vi "TL error.vi"(8 "error in (no error)":errorcluster, 11 "Return Code":i32) -> (0 "error out":errorcluster)   [LabVIEW 2014]
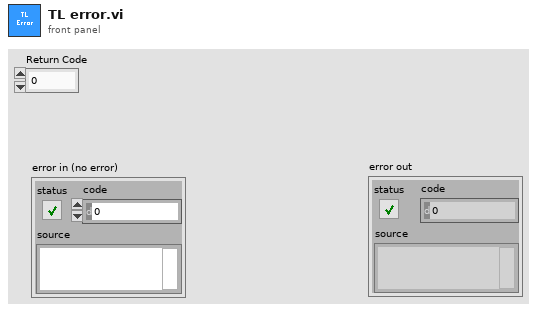
[diagram p1: front panel]
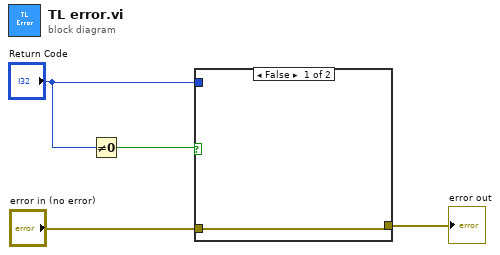
[diagram p0: block diagram]
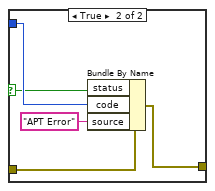
[diagram p2: hidden frame]
diagram:
  n1 = Not Equal To 0?(x="Return Code") -> (x != 0?=w3:bool)
  n2 = case shown="False" w3 {
    selector: w3 -> [_ w8]
    tunnel: "Return Code" -> [_ w9]
    tunnel: "error in (no error)" -> [w5 w10]
    tunnel: [w5 w6] -> w1
    frame False {
    }
    frame True {
      n3 = Bundle By Name(cluster=w10, "status"=w8, "code"=w9, "source"="APT Error") -> (w6:errorcluster)
    }
  }
  "error out" <- w1
